vi "Periodic Tasks.vi"(8 "error in":errorcluster) -> ()   [LabVIEW 2025]
doc: "This VI runs in parallel to other tasks. It can contain as many user-defined periodic loops as you need. These can carry out PID or other sorts of timed response."
uses:
  ButtonInfoTypeDef.ctl
  <vilib>/Utility/error.llb/Clear Errors.vi
  <vilib>/Rock Robotics/WPI/ThirdParty/JAS_Junk/TrajLib/VI/Util_GetTime_U32.vi
  <vilib>/Rock Robotics/WPI/ThirdParty/JAS_Junk/TrajLib/DigSeqLogic_On_Delay.vi
  <vilib>/Rock Robotics/WPI/ThirdParty/JAS_Junk/TrajLib/Timer_New.vi
  <vilib>/Rock Robotics/WPI/Utilities/WPI_GetSetVariantRefNum.vi
  Robot Global Data.vi
  <vilib>/Rock Robotics/SystemInterfaces/Utilities/FPGA_UtilitiesRead LocalTime.vi
  <vilib>/Rock Robotics/WPI/ThirdParty/JAS_Junk/TrajLib/VI/Util_GetTime_U64.vi
  <vilib>/Utility/semaphor.llb/Obtain Semaphore Reference.vi
  <vilib>/Rock Robotics/WPI/ThirdParty/JAS_Junk/TrajLib/Timer_Reset.vi
  <vilib>/Rock Robotics/WPI/ThirdParty/JAS_Junk/TrajLib/Timer_Start.vi
  <vilib>/Rock Robotics/WPI/ThirdParty/JAS_Junk/TrajLib/Timer_Stop.vi
  <vilib>/Rock Robotics/WPI/ThirdParty/JAS_Junk/TrajLib/Timer_HasPeriodPassedOnce.vi
  <vilib>/Rock Robotics/Network Tables/NT Read Boolean.vi
  <vilib>/Rock Robotics/Network Tables/NT Write Number.vi
  <vilib>/Rock Robotics/Network Tables/NT Write Boolean.vi
  <vilib>/Rock Robotics/WPI/ThirdParty/JAS_Junk/TrajLib/Trajectory_Library.lvlib
  <vilib>/Rock Robotics/WPI/ThirdParty/ChoreoLib/ChoreoLib.lvlib
panel:
  out "error out":errorcluster
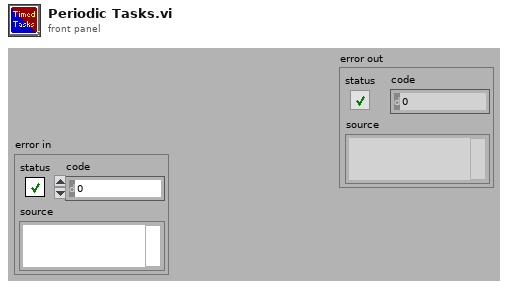
[diagram p1: front panel]
types:
  T1 = typedef "ButtonInfoTypeDef.ctl" = cluster{"ElapsedTime":dbl, "ButtonNumber":i32}
  T2 = typedef "WPI_JoystickDevRef.ctl" = cluster{"Device":T3}
  T3 = typedef "WPI_JoystickDeviceEnum.ctl" = enum16{"USB 0", "USB 1", "USB 2", "USB 3", "USB 4", "USB 5"}
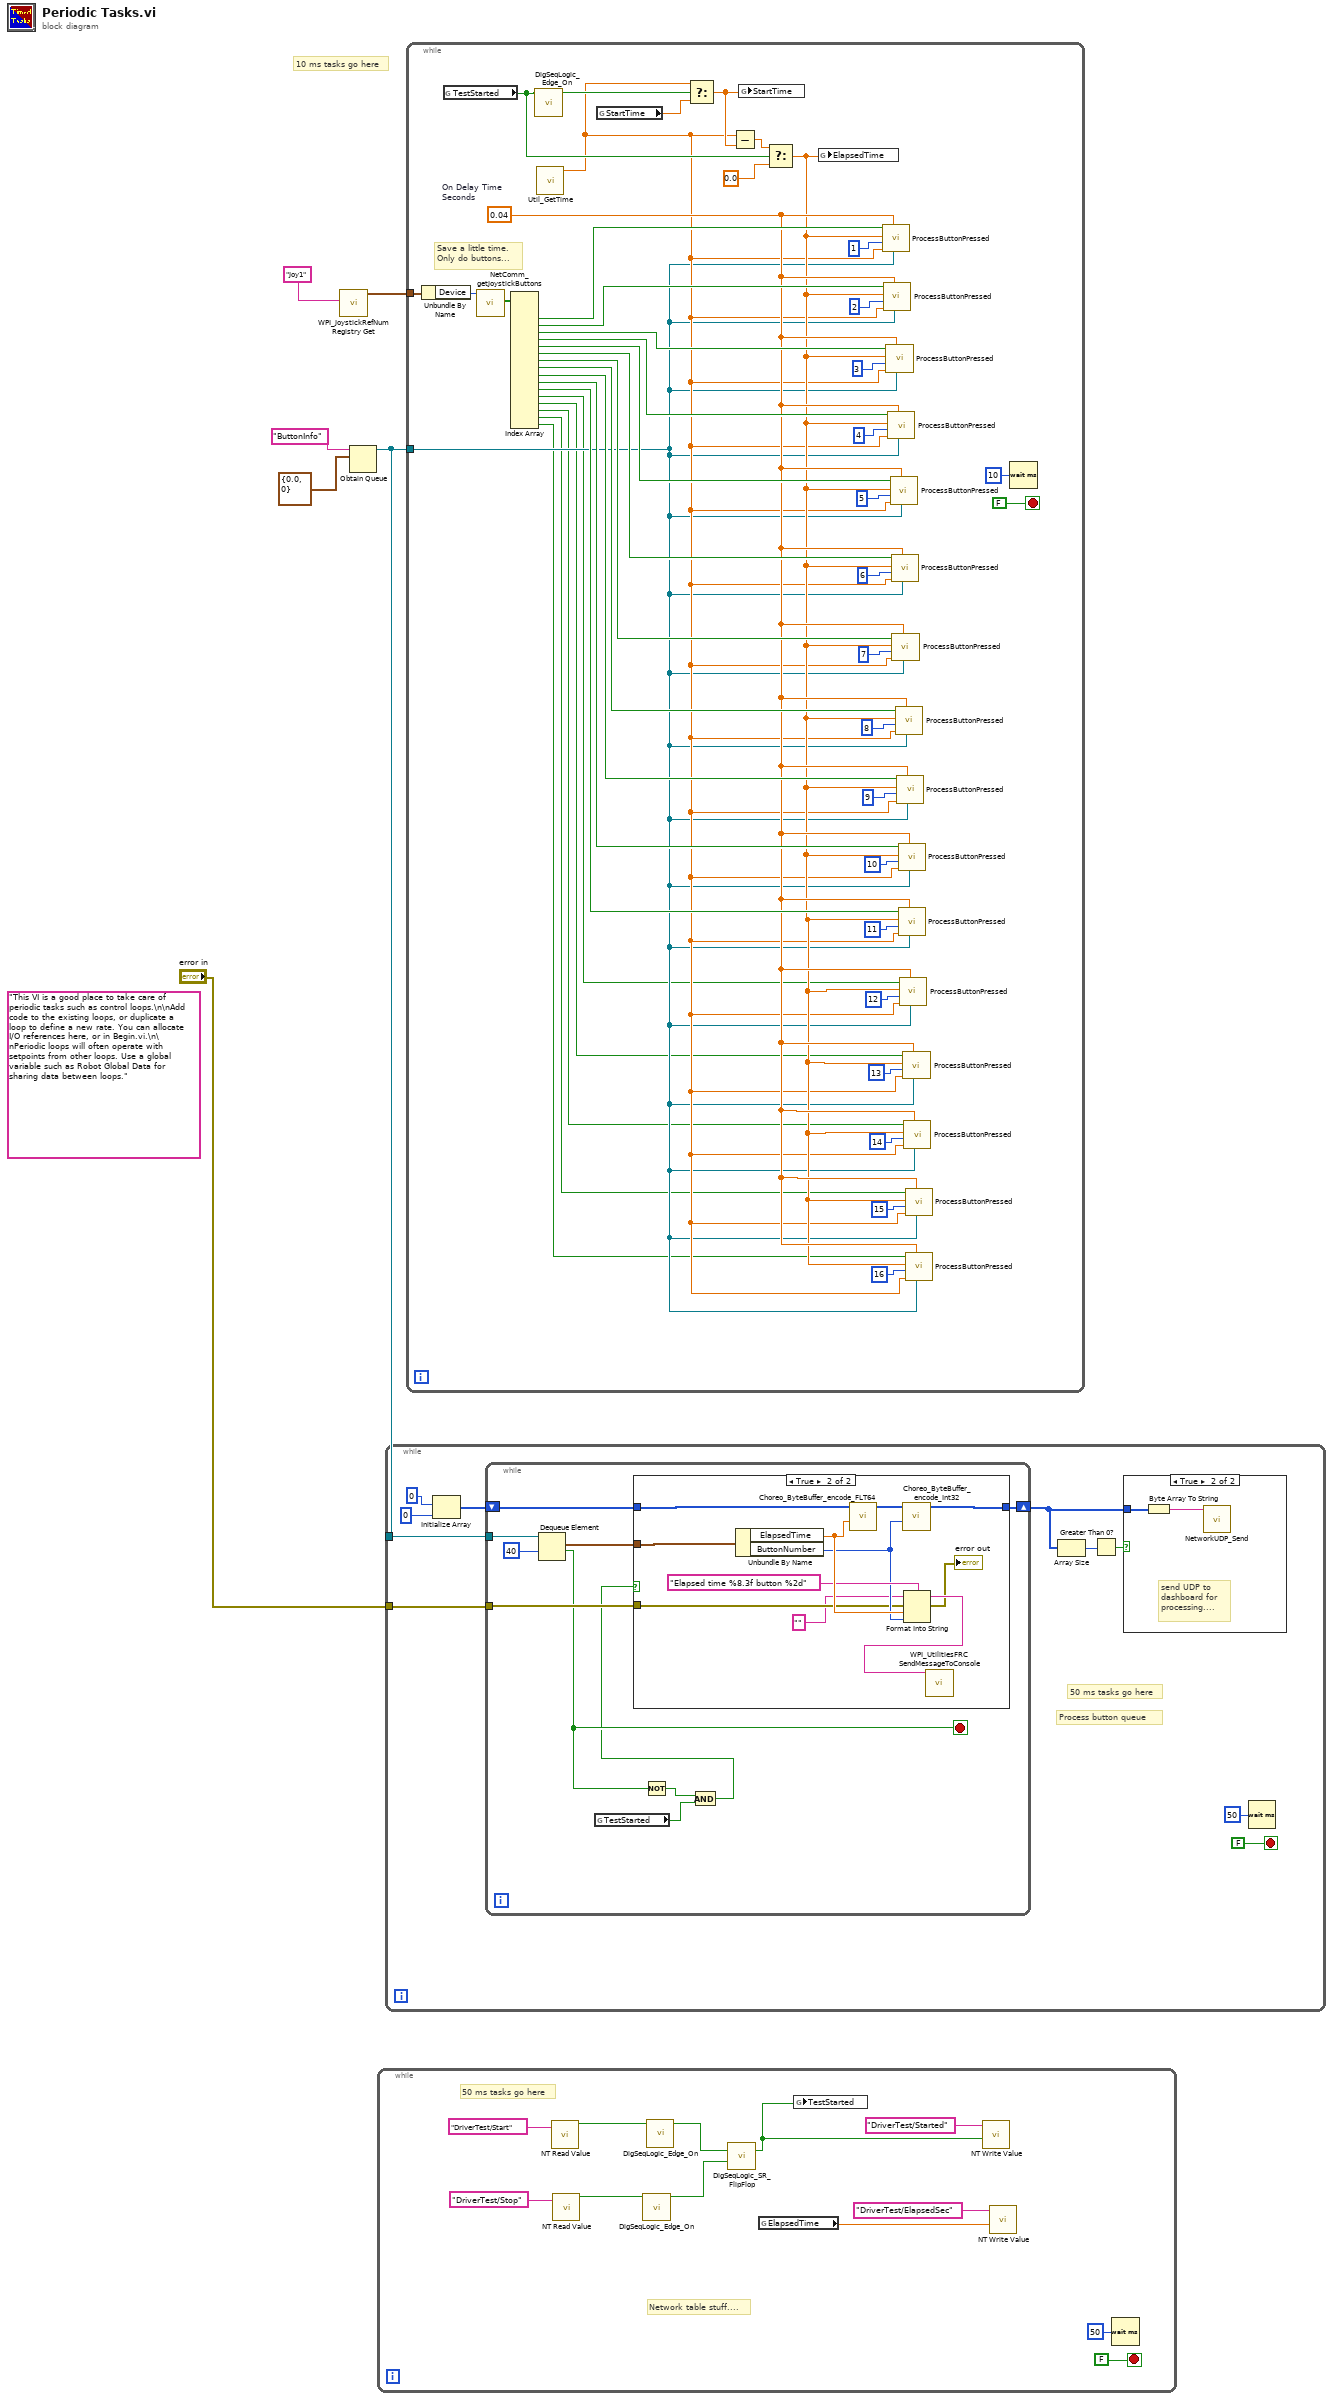
[diagram p0: block diagram]
diagram:
  (unwired) "This VI is a good place to take care of periodic tasks such as control loops.\n\nAdd code to the existing loops, or duplicate a loop to define a new rate. You can allocate I/O references here, or in Begin.vi.\n\nPeriodic loops will often operate with setpoints from other loops. Use a global variable such as Robot Global Data for sharing data between loops."
  # "10 ms tasks go here"
  n1 = call <vilib>:"WPI_JoystickRefNum Registry Get.vi"("refnum name"="Joy1") -> ("JoystickDevRef"=w5:T2)  [unwired: 1 in, 9 out]
  n2 = Obtain Queue(name (unnamed)="ButtonInfo", element data type=T1 {"ElapsedTime"=0.0, "ButtonNumber"=0} ("ButtonPressedInfo")) -> (queue out=w2:refnum<queue>)  [unwired: 3 in, 2 out]
  n3 = while {
    stop <- FALSE stop-if-true
    # "Network table stuff...."
    # "50 ms tasks go here"
    n4 = call-poly <vilib>:"NT Read Value.vi"("name"="DriverTest/Start") -> ("value"=w12:bool)  [unwired: 8 in, 2 out]
    n5 = call-poly <vilib>:"NT Read Value.vi"("name"="DriverTest/Stop") -> ("value"=w11:bool)  [unwired: 8 in, 2 out]
    n6 = call <vilib>:"DigSeqLogic_Edge_On.vi"("Input"=w11) -> ("On Edge"=w9:bool)  [unwired: 10 in]
    n7 = call <vilib>:"DigSeqLogic_Edge_On.vi"("Input"=w12) -> ("On Edge"=w10:bool)  [unwired: 10 in]
    n8 = call <vilib>:"DigSeqLogic_SR_FlipFlop.vi"("Set"=w10, "Reset"=w9) -> ("Output"=w8:bool)  [unwired: 12 in, 1 out]
    n9 = global read "Robot Global Data.vi" "ElapsedTime"() -> (w7:dbl)
    n10 = global write "Robot Global Data.vi" "TestStarted"(w8) -> ()
    n11 = call-poly <vilib>:"NT Write Value.vi"("value"=w8, "name"="DriverTest/Started") -> ()  [unwired: 9 in, 1 out]
    n12 = call-poly <vilib>:"NT Write Value.vi"("value"=w7, "name"="DriverTest/ElapsedSec") -> ()  [unwired: 9 in, 1 out]
    n13 = Wait (ms)(milliseconds to wait=u32 50) -> ()  [unwired: 1 out]
  }
  n14 = while {
    tunnel: w2 -> [w26]
    tunnel: "error in" -> [w19]
    stop <- FALSE stop-if-true
    # "Process button queue"
    # "50 ms tasks go here"
    n15 = Initialize Array(u8 0 ("Byte"), 0 ("dimension size")) -> (w23:u8[])
    n16 = while {
      tunnel: w26 -> [w40]
      shift-right: [w36] -> w22
      shift-left: w23 -> [w37]
      tunnel: w19 -> [w35]
      stop <- w32 stop-if-true
      n17 = Dequeue Element(queue=w40, timeout in ms (-1)=40) -> (element=w38:T1, timed out?=w32:bool)  [unwired: 1 in, 2 out]
      n18 = global read "Robot Global Data.vi" "TestStarted"() -> (w33:bool)
      n19 = Not(x=w32) -> (.not. x?=w34:bool)
      n20 = And(x=w34, y=w33) -> (x .and. y?=w31:bool)
      n21 = case shown="True" w31 {
        tunnel: w38 -> [_ w52]
        tunnel: w37 -> [w41 w51]
        tunnel: [w41 w49] -> w36
        tunnel: w35 -> [_ w43]
        frame False {
        }
        frame True {
          n22 = Unbundle By Name(w52) -> ("ElapsedTime"=w48:dbl, "ButtonNumber"=w46:i32)
          n23 = call <vilib>:"Choreo_ByteBuffer_encode_FLT64.vi"("FLT64_Value"=w48, "RawData In"=w51) -> ("RawData Out"=w50:u8[])  [unwired: 9 in]
          n24 = call <vilib>:"Choreo_ByteBuffer_encode_Int32.vi"("Int32_Value"=w46, "RawData In"=w50) -> ("RawData Out"=w49:u8[])  [unwired: 9 in]
          n25 = Format Into String(format string="Elapsed time %8.3f button %2d", initial string="", error in=w43, w48, w46) -> (resulting string=w45:string, error out=→"error out":errorcluster)
          n26 = call <vilib>:"WPI_UtilitiesFRC SendMessageToConsole.vi"("Message"=w45) -> ()  [unwired: 14 in, 1 out]
        }
      }
    }
    n27 = Array Size(array=w22) -> (size(s)=w21:i32)
    n28 = Greater Than 0?(x=w21) -> (x > 0?=w20:bool)
    n29 = case shown="True" w20 {
      tunnel: w22 -> [_ w30]
      frame False {
      }
      frame True {
        # "send UDP to \ndashboard for \nprocessing...."
        n30 = Byte Array To String(unsigned byte array=w30) -> (string=w29:string)
        n31 = call <vilib>:"NetworkUDP_Send.vi"("data string"=w29) -> ()  [unwired: 7 in, 4 out]
      }
    }
    n32 = Wait (ms)(milliseconds to wait=u32 50) -> ()  [unwired: 1 out]
  }
  n33 = while {
    tunnel: w5 -> [w97]
    tunnel: w2 -> [w58]
    stop <- FALSE stop-if-true
    w61 = 0.04  # On Delay Time Seconds
    # "Save a little time.\nOnly do buttons..."
    n34 = Unbundle By Name(w97) -> ("Device"=w96:T3)
    n35 = global read "Robot Global Data.vi" "TestStarted"() -> (w92:bool)
    n36 = call <vilib>:"NetComm_getJoystickButtons.vi"("Joystick Number"=w96) -> ("Buttons"=w95:bool[])  [unwired: 9 in, 1 out]
    n37 = Index Array(array=w95) -> (element #2=w87:bool, element #3=w82:bool, element #4=w81:bool, element #5=w80:bool, element #6=w79:bool, element #7=w72:bool, element #8=w71:bool, element #9=w70:bool, element #10=w69:bool, element #11=w68:bool, element #12=w67:bool, element #13=w57:bool, element #14=w56:bool, element #15=w55:bool, element #16=w54:bool, element #17=w53:bool)  [unwired: 17 in, 1 out]
    n38 = call <vilib>:"DigSeqLogic_Edge_On.vi"("Input"=w92) -> ("On Edge"=w94:bool)  [unwired: 10 in]
    n39 = call <vilib>:"Util_GetTime.vi"() -> ("FPGA_Time_Seconds"=w59:dbl)  [unwired: 9 in, 2 out]
    n40 = global read "Robot Global Data.vi" "StartTime"() -> (w93:dbl)
    n41 = Select(t=w59, s=w94, f=w93) -> (s? t:f=w89:dbl)
    n42 = Subtract(x=w59, y=w89) -> (x-y=w90:dbl)
    n43 = global write "Robot Global Data.vi" "StartTime"(w89) -> ()
    n44 = Select(t=w90, s=w92, f=0.0) -> (s? t:f=w60:dbl)
    n45 = global write "Robot Global Data.vi" "ElapsedTime"(w60) -> ()
    n46 = call "ProcessButtonPressed.vi"("Queue in"=w58, "On Delay Time\nSeconds"=w61, "Time"=w59, "ButtonNumber"=1, "ElapsedTime"=w60, "RawButtonInput"=w87) -> ()  [unwired: 6 in]
    n47 = call "ProcessButtonPressed.vi"("Queue in"=w58, "On Delay Time\nSeconds"=w61, "Time"=w59, "ButtonNumber"=2, "ElapsedTime"=w60, "RawButtonInput"=w82) -> ()  [unwired: 6 in]
    n48 = call "ProcessButtonPressed.vi"("Queue in"=w58, "On Delay Time\nSeconds"=w61, "Time"=w59, "ButtonNumber"=3, "ElapsedTime"=w60, "RawButtonInput"=w81) -> ()  [unwired: 6 in]
    n49 = call "ProcessButtonPressed.vi"("Queue in"=w58, "On Delay Time\nSeconds"=w61, "Time"=w59, "ButtonNumber"=4, "ElapsedTime"=w60, "RawButtonInput"=w80) -> ()  [unwired: 6 in]
    n50 = call "ProcessButtonPressed.vi"("Queue in"=w58, "On Delay Time\nSeconds"=w61, "Time"=w59, "ButtonNumber"=5, "ElapsedTime"=w60, "RawButtonInput"=w79) -> ()  [unwired: 6 in]
    n51 = call "ProcessButtonPressed.vi"("Queue in"=w58, "On Delay Time\nSeconds"=w61, "Time"=w59, "ButtonNumber"=6, "ElapsedTime"=w60, "RawButtonInput"=w72) -> ()  [unwired: 6 in]
    n52 = call "ProcessButtonPressed.vi"("Queue in"=w58, "On Delay Time\nSeconds"=w61, "Time"=w59, "ButtonNumber"=7, "ElapsedTime"=w60, "RawButtonInput"=w71) -> ()  [unwired: 6 in]
    n53 = call "ProcessButtonPressed.vi"("Queue in"=w58, "On Delay Time\nSeconds"=w61, "Time"=w59, "ButtonNumber"=8, "ElapsedTime"=w60, "RawButtonInput"=w70) -> ()  [unwired: 6 in]
    n54 = call "ProcessButtonPressed.vi"("Queue in"=w58, "On Delay Time\nSeconds"=w61, "Time"=w59, "ButtonNumber"=9, "ElapsedTime"=w60, "RawButtonInput"=w69) -> ()  [unwired: 6 in]
    n55 = call "ProcessButtonPressed.vi"("Queue in"=w58, "On Delay Time\nSeconds"=w61, "Time"=w59, "ButtonNumber"=10, "ElapsedTime"=w60, "RawButtonInput"=w68) -> ()  [unwired: 6 in]
    n56 = call "ProcessButtonPressed.vi"("Queue in"=w58, "On Delay Time\nSeconds"=w61, "Time"=w59, "ButtonNumber"=11, "ElapsedTime"=w60, "RawButtonInput"=w67) -> ()  [unwired: 6 in]
    n57 = call "ProcessButtonPressed.vi"("Queue in"=w58, "On Delay Time\nSeconds"=w61, "Time"=w59, "ButtonNumber"=12, "ElapsedTime"=w60, "RawButtonInput"=w57) -> ()  [unwired: 6 in]
    n58 = call "ProcessButtonPressed.vi"("Queue in"=w58, "On Delay Time\nSeconds"=w61, "Time"=w59, "ButtonNumber"=13, "ElapsedTime"=w60, "RawButtonInput"=w56) -> ()  [unwired: 6 in]
    n59 = call "ProcessButtonPressed.vi"("Queue in"=w58, "On Delay Time\nSeconds"=w61, "Time"=w59, "ButtonNumber"=14, "ElapsedTime"=w60, "RawButtonInput"=w55) -> ()  [unwired: 6 in]
    n60 = call "ProcessButtonPressed.vi"("Queue in"=w58, "On Delay Time\nSeconds"=w61, "Time"=w59, "ButtonNumber"=15, "ElapsedTime"=w60, "RawButtonInput"=w54) -> ()  [unwired: 6 in]
    n61 = call "ProcessButtonPressed.vi"("Queue in"=w58, "On Delay Time\nSeconds"=w61, "Time"=w59, "ButtonNumber"=16, "ElapsedTime"=w60, "RawButtonInput"=w53) -> ()  [unwired: 6 in]
    n62 = Wait (ms)(milliseconds to wait=u32 10) -> ()  [unwired: 1 out]
  }
